vi "factorial.vi"(8 "error in (no error)":errorcluster, 11 "n":i32) -> (0 "error out":errorcluster, 3 "n!":i32)   [LabVIEW 2020]
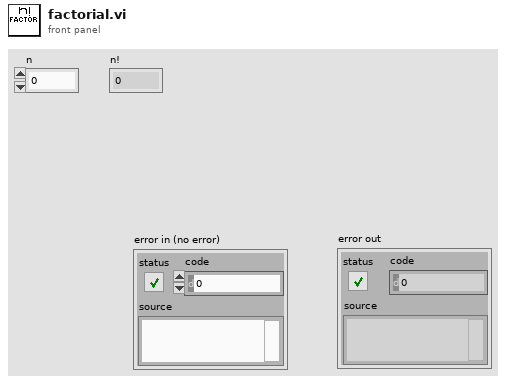
[diagram p1: front panel]
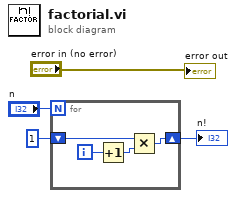
[diagram p0: block diagram]
diagram:
  n1 = for {
    N: "n" -> [_]
    shift-right: [w5] -> w2
    shift-left: 1 -> [w7]
    i -> [w8]
    n2 = Increment(x=w8) -> (x+1=w6:i32)
    n3 = Multiply(x=w7, y=w6) -> (x*y=w5:i32)
  }
  "n!" <- w2
  "error out" <- "error in (no error)"
